vi "sc5511a_list_buffer_write.vi"(0 "deviceHandle":u32 format="%.0x", 2 "List Frequency":u64=100000000 max=6500000000 format="%#.9p", 5 "error in":errorcluster) -> (14 "deviceHandle":u32 format="%.0x", 19 "error out":errorcluster)   [LabVIEW 2010]
uses:
  sc5511a.dll
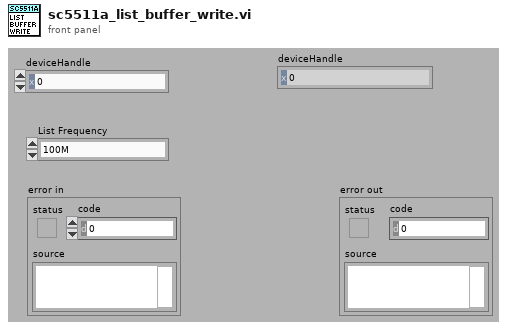
[diagram p1: front panel]
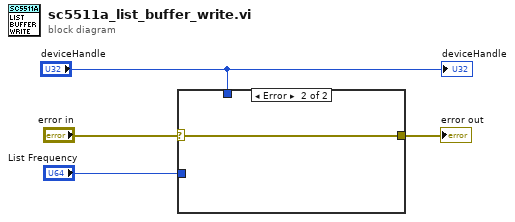
[diagram p0: block diagram]
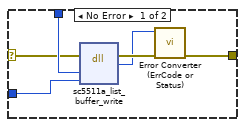
[diagram p2: hidden frame]
diagram:
  n1 = case shown="Error" "error in" {
    selector: "error in" -> [w5 w11]
    tunnel: [w10 w11] -> w4
    tunnel: "deviceHandle" -> [w7 _]
    tunnel: "List Frequency" -> [w6 _]
    frame No Error {
      n2 = dll-call lib="sc5511a.dll" fn="sc5511a_list_buffer_write"(error in=w5, "deviceHandle"=w7, "Frequency"=w6) -> (error out=w9:errorcluster, "return type"=w8:i32)  [unwired: 4 in, 1 out]
      n3 = call "Error Converter (ErrCode or Status).vi"("error in (no error)"=w9, "error code"=w8) -> ("error out"=w10:errorcluster)  [unwired: 9 in]
    }
    frame Error {
    }
  }
  "error out" <- w4
  "deviceHandle" <- "deviceHandle"
